vi "Finish Scan.vi"(8 "error in (no error)":errorcluster, 11 "Scanner in":refnum<class "Scanner.lvclass">) -> (0 "error out":errorcluster, 3 "Scanner out":refnum<class "Scanner.lvclass">)   [LabVIEW 2009, in "Scanner.lvclass"]
doc: "(Dynamic) Perform any cleanup after the last step. Restore the instrument to its initial pre-scan state if \"Return to Start\" is true."
uses:
  Scanner.lvclass
  Scanner.lvclass/Scanner.ctl
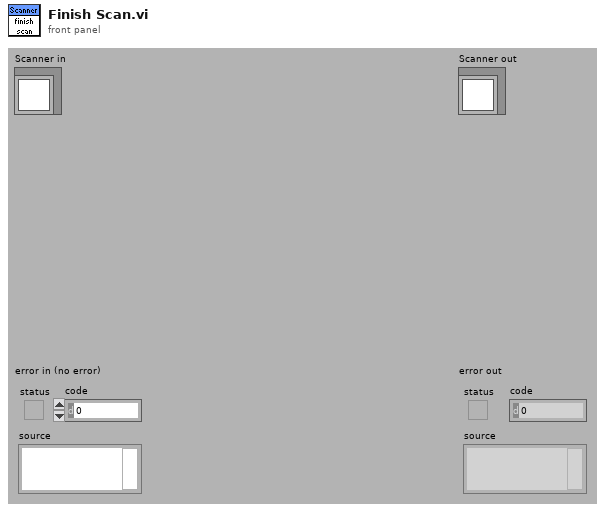
[diagram p1: front panel]
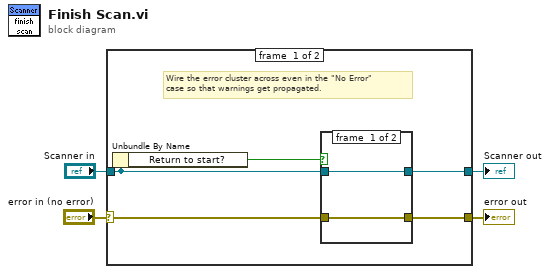
[diagram p0: block diagram]
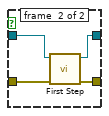
[diagram p2: hidden frame]
diagram:
  n1 = case shown="No Error" "error in (no error)" {
    selector: "error in (no error)" -> [w6 w17]
    tunnel: [w5 w17] -> w3
    tunnel: [w7 w16] -> w1
    tunnel: "Scanner in" -> [w8 w16]
    frame #0 {
      # "Wire the error cluster across even in the \"No Error\"\ncase so that warnings get propagated."
      n2 = Unbundle By Name(w8) -> ("Return to start?"=w9:bool)
      n3 = case shown="True" w9 {
        tunnel: w6 -> [w10 w15]
        tunnel: w8 -> [w11 w14]
        tunnel: [w11 w13] -> w7
        tunnel: [w10 w12] -> w5
        frame #0 {
        }
        frame #1 {
          n4 = call-dynamic "First Step.vi"("error in (no error)"=w15, "Scanner.lvclass in"=w14) -> ("error out"=w12:errorcluster, "Scanner.lvclass out"=w13:refnum<class "Scanner.lvclass">)  [unwired: 8 out]
        }
      }
    }
    frame #1 {
    }
  }
  "error out" <- w3
  "Scanner out" <- w1
